vi "Replace word with int.vi"(10 "Cluster":T1, 11 "String in":string) -> (3 "String out":string)   [LabVIEW 2020, in "Words to Numbers Converter.lvclass"]
uses:
  Words to Numbers Converter.lvclass
  Word in String.ctl
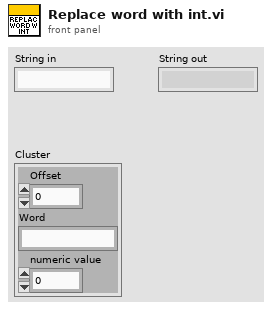
[diagram p1: front panel]
types:
  T1 = typedef "Words to Numbers Converter.lvclass/Word in String.ctl" = cluster{"Offset":i32, "Word":string, "numeric value":i32}
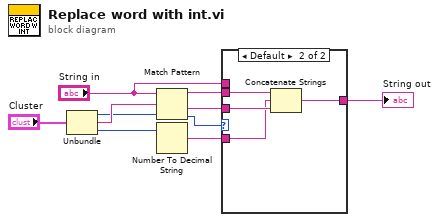
[diagram p0: block diagram]
diagram:
  n1 = Unbundle("Cluster") -> ("Offset"=w4:i32, "Word"=w7:string, "numeric value"=w3:i32)
  n2 = Match Pattern(string="String in", regular expression=w7, offset (0)=w4) -> (before substring=w8:string, after substring=w9:string, offset past match=w2:i32)  [unwired: 1 out]
  n3 = Number To Decimal String(number=w3) -> (decimal integer string=w6:string)  [unwired: 1 in]
  n4 = case shown="Default" w2 {
    tunnel: [w11 w15] -> w10
    tunnel: w9 -> [_ w14]
    tunnel: w8 -> [_ w13]
    tunnel: w6 -> [_ w12]
    tunnel: "String in" -> [w11 _]
    frame -1 {
    }
    frame Default {
      n5 = Concatenate Strings(w13, w12, w14) -> (w15:string)
    }
  }
  "String out" <- w10
